vi "RegisterWindow.vi"(8 "error in (no error)":errorcluster, 10 "Window":refnum<class "Window.lvclass">, 11 "Engine in":refnum<class "Engine.lvclass">) -> (0 "error out":errorcluster, 3 "Engine out":refnum<class "Engine.lvclass">)   [LabVIEW 2024, in "GLF.lvlib" / "Engine.lvclass"]
uses:
  Engine.lvclass
  Window/Window.lvclass
  Engine.lvclass/Engine.ctl
  Command--enum.ctl
  Command-RegisterWindow--cluster.ctl
  C:/Users/Thomas/Documents/Projects/GLF/Sources/GLF/IUseDVRHandler/IUseDVRHandler.lvclass
  C:/Users/Thomas/Documents/Projects/GLF/Sources/GLF/IAmGLF/IAmGLF.lvclass
  C:/Users/Thomas/Documents/Projects/GLF/Sources/GLF/Window/Window.lvclass
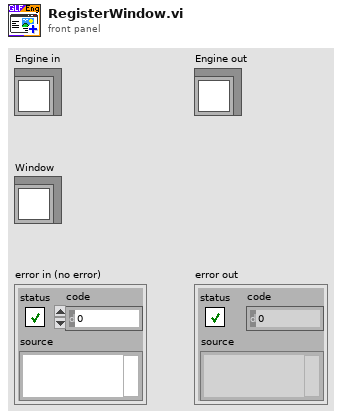
[diagram p1: front panel]
types:
  T1 = typedef "GLF.lvlib/Engine.lvclass/Command-RegisterWindow--cluster.ctl" = cluster{"Window":refnum<class "Window.lvclass">, "Error Return Notifier":refnum<notifier>}
  T2 = typedef "GLF.lvlib/Engine.lvclass/Command--enum.ctl" = enum16{"Quit", "Create DVR", "Delete DVR", "Register Window"}
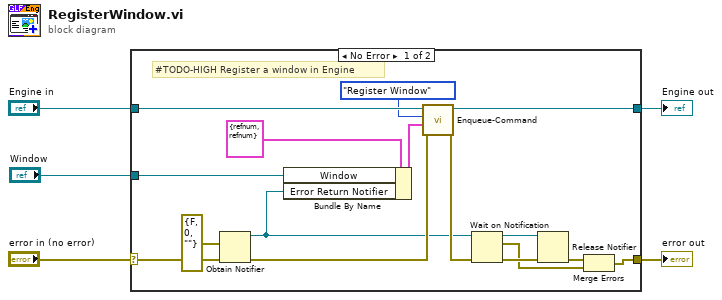
[diagram p0: block diagram]
diagram:
  n1 = case shown="No Error" "error in (no error)" {
    selector: "error in (no error)" -> [w13 w23]
    tunnel: [w7 w23] -> w4
    tunnel: [w20 w22] -> w2
    tunnel: "Engine in" -> [w21 w22]
    tunnel: "Window" -> [w9 _]
    frame No Error {
      # "#TODO-HIGH Register a window in Engine"
      n2 = Obtain Notifier(notification data type=errorcluster {"status"=FALSE, "code"=0, "source"=""} ("error in (no error)"), error in (no error)=w13) -> (notifier out=w8:refnum<notifier>, error out=w15:errorcluster)  [unwired: 2 in, 1 out]
      n3 = Bundle By Name(cluster=T1 {"Window"=refnum, "Error Return Notifier"=refnum} ("Data"), "Window"=w9, "Error Return Notifier"=w8) -> (w10:T1)
      n4 = call "Enqueue-Command.vi"("error in (no error)"=w15, "Cmd Data"=w10, "Cmd"=Command--enum."Register Window", "Engine in"=w21) -> ("error out"=w14:errorcluster, "Engine out"=w20:refnum<class "Engine.lvclass">)  [unwired: 5 in, 1 out]
      n5 = Wait on Notification(notifier=w8, error in (no error)=w14) -> (notifier out=w16:refnum<notifier>, notification=w6:errorcluster, error out=w18:errorcluster)  [unwired: 2 in, 1 out]
      n6 = Release Notifier(notifier=w16, error in (no error)=w18) -> (error out=w12:errorcluster)  [unwired: 1 in, 2 out]
      n7 = Merge Errors(w12, w6) -> (w7:errorcluster)
    }
    frame Error {
    }
  }
  "error out" <- w4
  "Engine out" <- w2
